vi "lock.vi"(8 "error in":errorcluster, 10 "password":string, 11 "connection ID":refnum<k5>) -> (0 "error out":errorcluster, 3 "connection ID":refnum<k5>)   [LabVIEW 2016]
panel:
  in  "Set Command":string="lock"
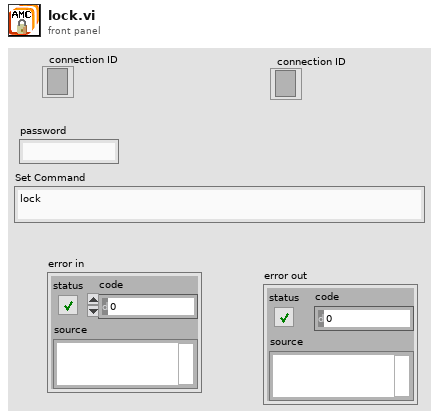
[diagram p1: front panel]
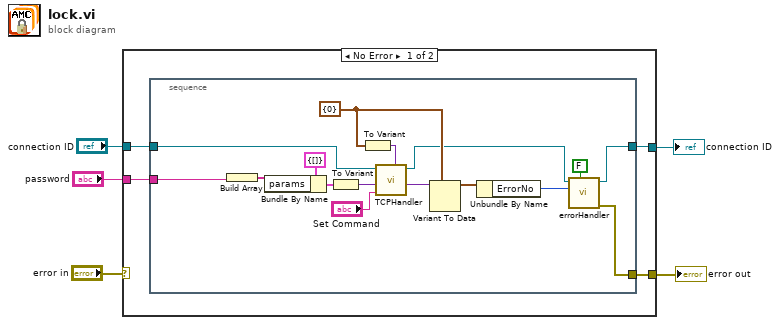
[diagram p0: block diagram]
diagram:
  n1 = case shown="No Error" "error in" {
    selector: "error in" -> [_ w26]
    tunnel: [w6 w26] -> w5
    tunnel: [w7 w27] -> w4
    tunnel: "connection ID" -> [w8 w27]
    tunnel: "password" -> [w9 _]
    frame No Error {
      n2 = stacked-sequence {
        tunnel: [w10] -> w7
        tunnel: w8 -> [w16]
        tunnel: [w17] -> w6
        tunnel: w9 -> [w12]
        frame #0 {
          w14 = cluster{"ErrorNo":i32} {"ErrorNo"=0} ("input cluster")
          n3 = Build Array(w12) -> (w21:string[])
          n4 = Bundle By Name(cluster=cluster{"params":string[]} {"params"=[]} ("input cluster"), "params"=w21) -> (w22:cluster{"params":string[]})
          n5 = To Variant(anything=w22) -> (Variant=w23:variant)
          n6 = To Variant(anything=w14) -> (Variant=w15:variant)
          n7 = call "TCPHandler.vi"("result Types"=w15, "method"="Set Command", "params"=w23, "connection ID"=w16) -> ("result"=w19:variant, "connection ID"=w11:refnum<k5>)  [unwired: 5 in, 1 out]
          n8 = Variant To Data(type=w14, Variant=w19) -> (data=w24:cluster{"ErrorNo":i32})  [unwired: 1 in, 1 out]
          n9 = Unbundle By Name(w24) -> ("ErrorNo"=w25:i32)
          n10 = call "errorHandler.vi"("show popup"=FALSE, "error number"=w25, "connection ID"=w11) -> ("error out"=w17:errorcluster, "connection ID"=w10:refnum<k5>)  [unwired: 7 in]
        }
      }
    }
    frame Error {
    }
  }
  "error out" <- w5
  "connection ID" <- w4
